vi "CreateAppConfig.vi"(8 "error in":errorcluster) -> (0 "error out":errorcluster)   [LabVIEW 2020, in "ORM_API.lvlib"]
doc: "Creates the app.config file if it doesn't already exist.\nThis file is written next to the lvproj if in development mode\nThis file is written next to the EXE if executed in the runtime\n\nNOTE: If the EXE resides in a protected location, the the application may need to be launched as an administrator"
uses:
  ORM_API.lvlib
  <vilib>/Utility/error.llb/Error Cluster From Error Code.vi
  <vilib>/ErrorRing/Error Ring.xnode
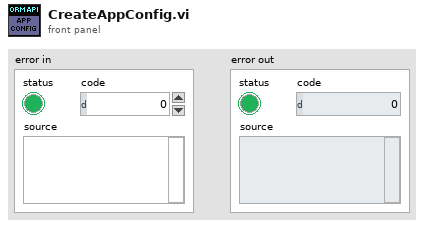
[diagram p1: front panel]
types:
  T1 = enum16{"open", "replace", "create", "open or create", "replace or create", "replace or create with confirmation"}
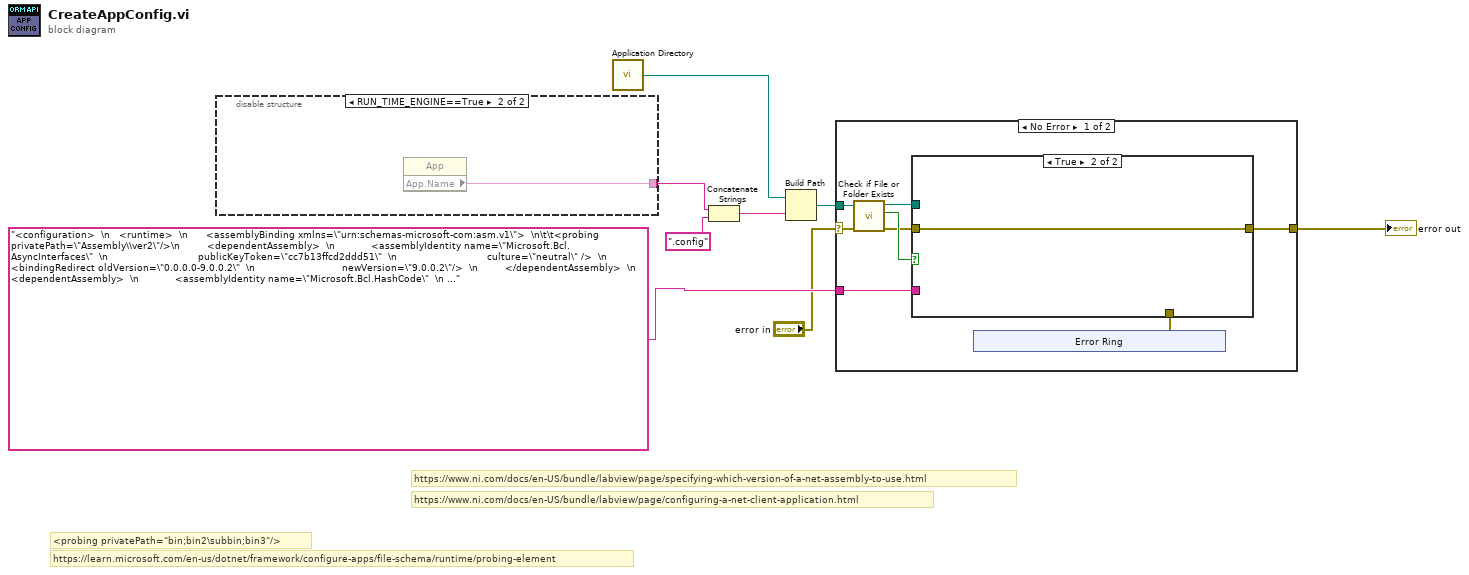
[diagram p0: block diagram]
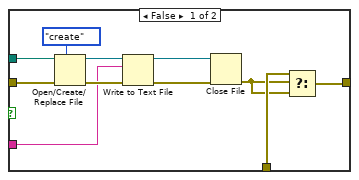
[diagram p2: hidden frame]
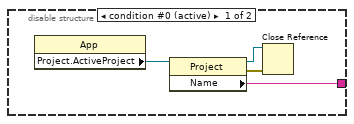
[diagram p4: hidden frame]
diagram:
  # "https://www.ni.com/docs/en-US/bundle/labview/page/specifying-which-version-of-a-net-assembly-to-use.html"
  # "https://learn.microsoft.com/en-us/dotnet/framework/configure-apps/file-schema/runtime/probing-element"
  # "<probing privatePath=\"bin;bin2\\subbin;bin3\"/>"
  # "https://www.ni.com/docs/en-US/bundle/labview/page/configuring-a-net-client-application.html"
  n1 = disable-structure shown="RUN_TIME_ENGINE==True" {
    disable-tunnel: [w11 w13] -> w8
    frame condition #0 (active) {
      n2 = property class="App"() -> ("Project.ActiveProject"=w12:refnum<vi>)  [unwired: 2 in, 2 out]
      n3 = property class="Project"(reference=w12) -> (reference out=w10:refnum<vi>, error out=w9:errorcluster, "Name"=w11:string)  [unwired: 1 in]
      n4 = Close Reference(reference=w10, error in (no error)=w9) -> ()  [unwired: 1 out]
    }
    frame condition #1 {
      n5 = property class="App"() -> ("App.Name"=w13:string)  [unwired: 2 in, 2 out]
    }
  }
  n6 = call <vilib>:"Application Directory.vi"() -> ("Application Directory"=w5:path)
  n7 = Concatenate Strings(w8, ".config" ("string")) -> (w6:string)
  n8 = Build Path(base path=w5, name or relative path=w6) -> (appended path=w4:path)
  n9 = case shown="No Error" "error in" {
    selector: "error in" -> [w14 w39]
    tunnel: w4 -> [w21 _]
    tunnel: "<configuration>  \n   <runtime>  \n      <assemblyBinding xmlns=\"urn:schemas-microsoft-com:asm.v1\">  \n\t\t<probing privatePath=\"Assembly\\ver2\"/>\n         <dependentAssembly>  \n            <assemblyIdentity name=\"Microsoft.Bcl.AsyncInterfaces\"  \n                              publicKeyToken=\"cc7b13ffcd2ddd51\"  \n                              culture=\"neutral\" />  \n            <bindingRedirect oldVersion=\"0.0.0.0-9.0.0.2\"  \n                             newVersion=\"9.0.0.2\"/>  \n         </dependentAssembly>  \n         <dependentAssembly>  \n            <assemblyIdentity name=\"Microsoft.Bcl.HashCode\"  \n                              publicKeyToken=\"cc7b13ffcd2ddd51\"  \n                              culture=\"neutral\" />  \n            <bindingRedirect oldVersion=\"0.0.0.0-6.0.0.0\"  \n                             newVersion=\"6.0.0.0\"/>  \n         </dependentAssembly>   \n         <dependentAssembly>  \n            <assemblyIdentity name=\"Microsoft.Extensions.DependencyInjection.Abstractions\"  \n                              publicKeyToken=\"adb9793829ddae60\"  \n                              culture=\"neutral\" />  \n            <bindingRedirect oldVersion=\"0.0.0.0-9.0.0.0\"  \n                             newVersion=\"9.0.0.0\"/>  \n         </dependentAssembly>    \n         <dependentAssembly>  \n            <assemblyIdentity name=\"Microsoft.Extensions.Logging.Abstractions\"  \n                              publicKeyToken=\"adb9793829ddae60\"  \n                              culture=\"neutral\" />  \n            <bindingRedirect oldVersion=\"0.0.0.0-9.0.0.0\"  \n                             newVersion=\"9.0.0.0\"/>  \n         </dependentAssembly>     \n         <dependentAssembly>  \n            <assemblyIdentity name=\"Microsoft.IO.RecyclableMemoryStream\"  \n                              publicKeyToken=\"31bf3856ad364e35\"  \n                              culture=\"neutral\" />  \n            <bindingRedirect oldVersion=\"0.0.0.0-3.0.1.0\"  \n                             newVersion=\"3.0.1.0\"/>  \n         </dependentAssembly> \n         <dependentAssembly>  \n            <assemblyIdentity name=\"Pipelines.Sockets.Unofficial\"  \n                              publicKeyToken=\"42ea0a778e13fbe2\"  \n                              culture=\"neutral\" />  \n            <bindingRedirect oldVersion=\"0.0.0.0-1.0.0.0\"  \n                             newVersion=\"1.0.0.0\"/>  \n         </dependentAssembly>  \n         <dependentAssembly>  \n            <assemblyIdentity name=\"System.Buffers\"  \n                              publicKeyToken=\"cc7b13ffcd2ddd51\"  \n                              culture=\"neutral\" />  \n            <bindingRedirect oldVersion=\"0.0.0.0-4.0.2.0\"  \n                             newVersion=\"4.0.2.0\"/>  \n         </dependentAssembly> \n         <dependentAssembly>  \n            <assemblyIdentity name=\"System.Collections.Immutable\"  \n                              publicKeyToken=\"b03f5f7f11d50a3a\"  \n                              culture=\"neutral\" />  \n            <bindingRedirect oldVersion=\"0.0.0.0-9.0.0.0\"  \n                             newVersion=\"9.0.0.0\"/>  \n         </dependentAssembly>  \n         <dependentAssembly>  \n            <assemblyIdentity name=\"System.Diagnostics.DiagnosticSource\"  \n                              publicKeyToken=\"cc7b13ffcd2ddd51\"  \n                              culture=\"neutral\" />  \n            <bindingRedirect oldVersion=\"0.0.0.0-9.0.0.0\"  \n                             newVersion=\"9.0.0.0\"/>  \n         </dependentAssembly>   \n         <dependentAssembly>  \n            <assemblyIdentity name=\"System.IO.Pipelines\"  \n                              publicKeyToken=\"cc7b13ffcd2ddd51\"  \n                              culture=\"neutral\" />  \n            <bindingRedirect oldVersion=\"0.0.0.0-9.0.0.0\"  \n                             newVersion=\"9.0.0.0\"/>  \n         </dependentAssembly>    \n         <dependentAssembly>  \n            <assemblyIdentity name=\"System.Memory\"  \n                              publicKeyToken=\"cc7b13ffcd2ddd51\"  \n                              culture=\"neutral\" />  \n            <bindingRedirect oldVersion=\"0.0.0.0-4.0.2.0\"  \n                             newVersion=\"4.0.2.0\"/>  \n         </dependentAssembly>     \n         <dependentAssembly>  \n            <assemblyIdentity name=\"System.Numerics.Vectors\"  \n                              publicKeyToken=\"b03f5f7f11d50a3a\"  \n                              culture=\"neutral\" />  \n            <bindingRedirect oldVersion=\"0.0.0.0-4.1.3.0\"  \n                             newVersion=\"4.1.3.0\"/>  \n         </dependentAssembly>      \n         <dependentAssembly>  \n            <assemblyIdentity name=\"System.Reflection.Emit.ILGeneration\"  \n                              publicKeyToken=\"b03f5f7f11d50a3a\"  \n                              culture=\"neutral\" />  \n            <bindingRedirect oldVersion=\"0.0.0.0-4.0.0.0\"  \n                             newVersion=\"4.0.0.0\"/>  \n         </dependentAssembly>       \n         <dependentAssembly>  \n            <assemblyIdentity name=\"System.Reflection.Emit.Lightweight\"  \n                              publicKeyToken=\"b03f5f7f11d50a3a\"  \n                              culture=\"neutral\" />  \n            <bindingRedirect oldVersion=\"0.0.0.0-4.0.0.0\"  \n                             newVersion=\"4.0.0.0\"/>  \n         </dependentAssembly>        \n         <dependentAssembly>  \n            <assemblyIdentity name=\"System.Runtime.CompilerServices.Unsafe\"  \n                              publicKeyToken=\"b03f5f7f11d50a3a\"  \n                              culture=\"neutral\" />  \n            <bindingRedirect oldVersion=\"0.0.0.0-6.0.0.0\"  \n                             newVersion=\"6.0.0.0\"/>  \n         </dependentAssembly>         \n         <dependentAssembly>  \n            <assemblyIdentity name=\"System.Text.Encodings.Web\"  \n                              publicKeyToken=\"cc7b13ffcd2ddd51\"  \n                              culture=\"neutral\" />  \n            <bindingRedirect oldVersion=\"0.0.0.0-9.0.0.0\"  \n                             newVersion=\"9.0.0.0\"/>  \n         </dependentAssembly>          \n         <dependentAssembly>  \n            <assemblyIdentity name=\"System.Text.Json\"  \n                              publicKeyToken=\"cc7b13ffcd2ddd51\"  \n                              culture=\"neutral\" />  \n            <bindingRedirect oldVersion=\"0.0.0.0-9.0.0.0\"  \n                             newVersion=\"9.0.0.0\"/>  \n         </dependentAssembly>           \n         <dependentAssembly>  \n            <assemblyIdentity name=\"System.Threading.Channels\"  \n                              publicKeyToken=\"cc7b13ffcd2ddd51\"  \n                              culture=\"neutral\" />  \n            <bindingRedirect oldVersion=\"0.0.0.0-9.0.0.0\"  \n                             newVersion=\"9.0.0.0\"/>  \n         </dependentAssembly>            \n         <dependentAssembly>  \n            <assemblyIdentity name=\"System.Threading.Tasks.Extensions\"  \n                              publicKeyToken=\"cc7b13ffcd2ddd51\"  \n                              culture=\"neutral\" />  \n            <bindingRedirect oldVersion=\"0.0.0.0-4.2.1.0\"  \n                             newVersion=\"4.2.1.0\"/>  \n         </dependentAssembly> \n      </assemblyBinding>  \n   </runtime>  \n</configuration> " -> [w17 _]
    tunnel: [w15 w39] -> w2
    frame No Error {
      n10 = call <vilib>:"Check if File or Folder Exists.vi"("error in (no error)"=w14, "path"=w21) -> ("error out"=w18:errorcluster, "file or folder exists?"=w20:bool, "dup path"=w19:path)  [unwired: 7 in]
      n11 = xnode "Error Ring"() -> ("error out"=w16:errorcluster)
      n12 = case shown="True" w20 {
        tunnel: w19 -> [w37 _]
        tunnel: w18 -> [w36 w38]
        tunnel: w17 -> [w30 _]
        tunnel: w16 -> [w29 _]
        tunnel: [w27 w38] -> w15
        frame False {
          n13 = Open/Create/Replace File(file path (use dialog)=w37, error in=w36, operation (0:open)=T1."create") -> (refnum out=w34:refnum<file>, error out=w33:errorcluster)  [unwired: 3 in, 1 out]
          n14 = Write to Text File(file (use dialog)=w34, text=w30, error in=w33) -> (refnum out=w32:refnum<file>, error out=w31:errorcluster)  [unwired: 1 in, 1 out]
          n15 = Close File(refnum=w32, error in=w31) -> (error out=w28:errorcluster)  [unwired: 1 out]
          n16 = Select(t=w29, s=w28, f=w28) -> (s? t:f=w27:errorcluster)
        }
        frame True {
        }
      }
    }
    frame Error {
    }
  }
  "error out" <- w2
